vi "c_ctre_phoenix_report_error.vi"(0 "Numeric":i32, 1 "Numeric 2":i32, 2 "Numeric 3":i32, 3 "String 2":string, 4 "String 4":string, 5 "String 6":string) -> (20 "String":string, 21 "String 3":string, 22 "String 5":string)   [LabVIEW 2023]
uses:
  <vilib>/Rock Robotics/WPI/ThirdParty/Phoenix-LabVIEW/Controls/DriverLib.ctl
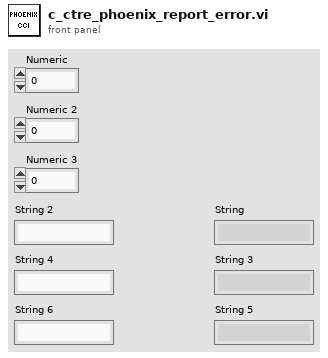
[diagram p1: front panel]
types:
  T1 = typedef "DriverLib.ctl" = path
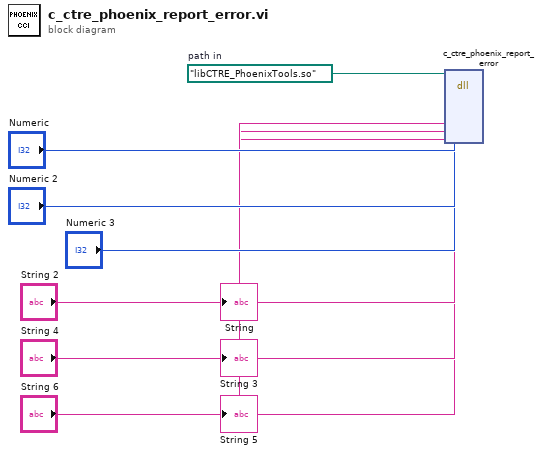
[diagram p0: block diagram]
diagram:
  w10 = T1 path "libCTRE_PhoenixTools.so"  # path in
  n1 = dll-call lib="?" fn="c_ctre_phoenix_report_error"(path in=w10, "Numeric", "Numeric 2", "Numeric 3", "String 2", "String 4", "String 6") -> (→"String":string, →"String 3":string, →"String 5":string)  [unwired: 6 in, 2 out]
